vi "Array2PyList.vi"(8 "error in (no error)":errorcluster caption="entrée d'erreur (pas d'erreur)", 11 "Tableau de valves":string[](array[string])=["08120001", "08120002", "08120003", "08120004"]) -> (0 "error out":errorcluster caption="sortie d'erreur", 3 "List_Valves":string=" 08120001,  08120002,  08120003,  08120004")   [LabVIEW 2020]
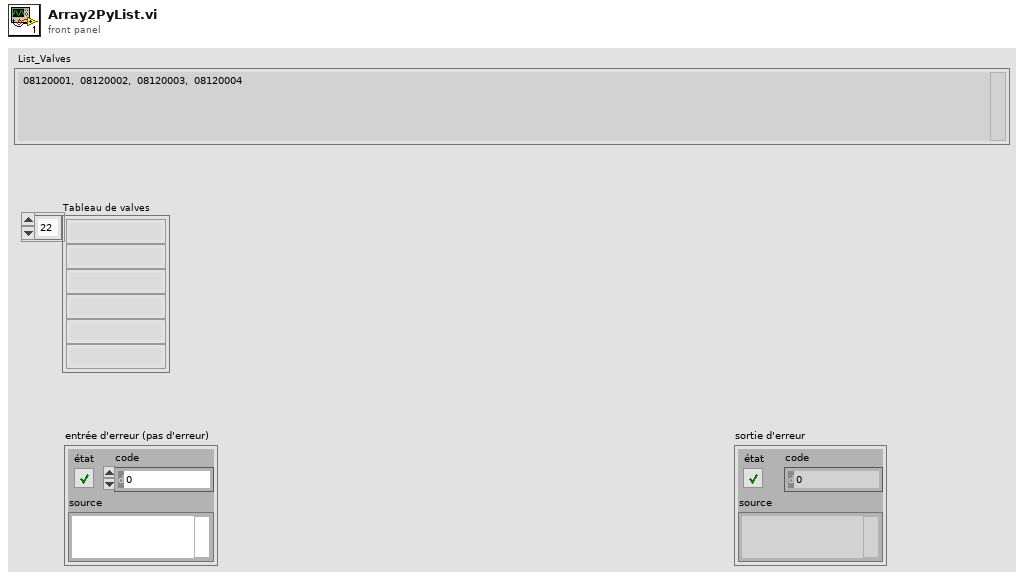
[diagram p1: front panel]
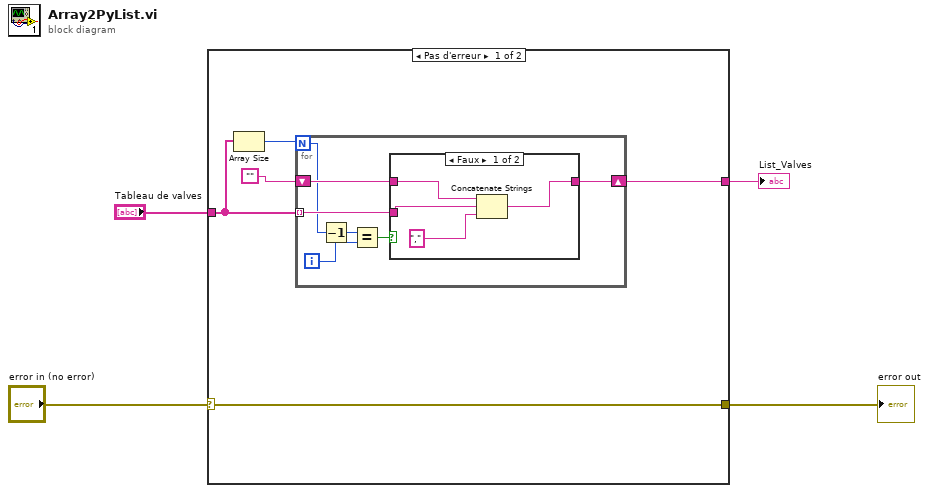
[diagram p0: block diagram]
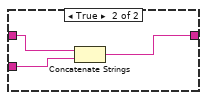
[diagram p2: hidden frame]
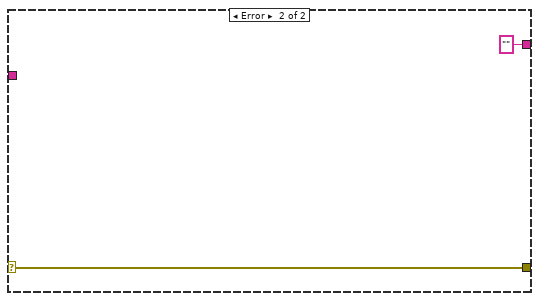
[diagram p3: hidden frame]
diagram:
  n1 = case shown="Pas d'erreur" "error in (no error)" {
    selector: "error in (no error)" -> [w5 w25]
    tunnel: "Tableau de valves" -> [w8 _]
    tunnel: [w6 ""] -> w3
    tunnel: [w5 w25] -> w1
    frame No Error {
      n2 = Array Size(array=w8) -> (size(s)=w9:i32)
      n3 = for {
        N: w9 -> [w12]
        tunnel: w8 -> [w15] mode=indexing
        shift-right: [w10] -> w6
        shift-left: "" -> [w16]
        i -> [w13]
        n4 = Decrement(x=w12) -> (x-1=w11:i32)
        n5 = Equal?(x=w11, y=w13) -> (x = y?=w14:bool)
        n6 = case shown="Faux" w14 {
          tunnel: w16 -> [w18 w21]
          tunnel: w15 -> [w20 w23]
          tunnel: [w19 w22] -> w10
          frame False {
            n7 = Concatenate Strings(w18, w20, ",") -> (w19:string)
          }
          frame True {
            n8 = Concatenate Strings(w21, w23) -> (w22:string)
          }
        }
      }
    }
    frame Error {
    }
  }
  "List_Valves" <- w3
  "error out" <- w1
